vi "SimulateLengthTF.vi"(5 "Numeric in":dbl, 6 "Cluster":cluster{"Weight":dbl, "Radius":dbl}, 7 "NumProcess":dbl[](array[numeric]), 8 "error in (no error)":errorcluster, 9 "Numeric 3":dbl, 10 "DenProces":dbl[](array[numeric]), 11 ".NET Refnum in":refnum<k24>) -> (0 "error out":errorcluster, 2 "Numeric out":dbl, 3 ".NET Refnum out":refnum<k24>)   [LabVIEW 2013]
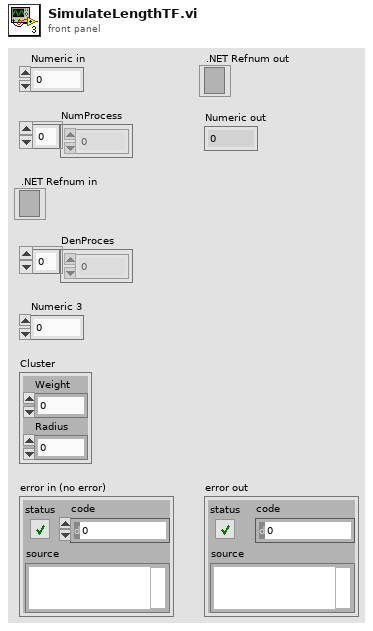
[diagram p1: front panel]
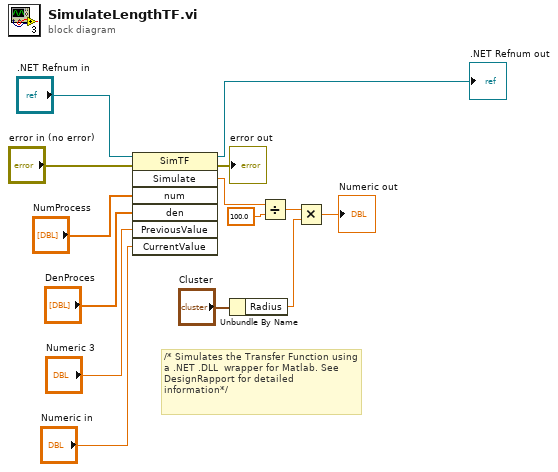
[diagram p0: block diagram]
diagram:
  # "/* Simulates the Transfer Function using a .NET .DLL  wrapper for Matlab. See DesignRapport for detailed information*/"
  n1 = invoke class="SimTF" method="Simulate"(reference=".NET Refnum in", error in="error in (no error)", "num"="NumProcess", "den"="DenProces", "PreviousValue"="Numeric 3", "CurrentValue"="Numeric in") -> (reference out=→".NET Refnum out":refnum<k24>, error out=→"error out":errorcluster, "Simulate"=w12:dbl)  [unwired: 1 in, 4 out]
  n2 = Unbundle By Name("Cluster") -> ("Radius"=w8:dbl)
  n3 = Divide(x=w12, y=100.0) -> (x/y=w13:dbl)
  n4 = Multiply(x=w13, y=w8) -> (x*y=→"Numeric out":dbl)
